vi "SDT_GenerateMeasureInfoBlockDecayCurves.vi"(4 "EndTimeArray":dbl[](array[numeric]), 8 "ActiveModule":string[](array[string]), 9 "DecayMatrix":u32[][](array[numeric]), 10 "Module Type":T12 items=["SPC-600"=600, "SPC-630"=630, "SPC-700"=700, "SPC-730"=730, "SPC-130"=130, "SPC-830"=830, "SPC-140"=140, "SPC-930"=930, "DPC-230"=230, "SPC-150"=150, "SPC-150 N"=151, "SPC-150 NX"=152, "SPC-130 EM"=131, "SPC-130 EMN"=132, "SPC-130IN"=135, "SPC-130INX"=136, "SPC-130INXX"=137, "SPC-160"=160, "SPC-160 X"=161, "SPC-160 PCIE"=162, "SPC-180 N"=180, "SPC-180 NX"=181, "SPC-180 NXX"=182, "SPC-180 N-USB"=185, "SPC-180 NX-USB"=186, "SPC-180 NXX-USB"=187, "SPC-QC-104"=104, "SPC-QC-004"=4, "SPC-QC-106"=106, "DPC-330"=330, "PMS-800"=800, "SPC-590"=590, "Simulation"=-1], 11 "SPCdata":T11[](array[typedef])) -> (2 "MeasureInfoStrings":string[](array[string]), 3 "MeasureInfos":T1[](array[typedef]) {"MeasStopInfo"."flags" format="x%x"})   [LabVIEW 2017]
doc: "This VI is a SubVI to SDT_WriteFile.vi. It populates the arrays of MeasureInfos cluster and generates strings ready to be written to file. \nFor a description of the *.sdt file format see: SPC_data_file_structure.h\n\ninfo@becker-hickl.com"
uses:
  SPC_Wrappers/SPC_Controls/ModuleType.ctl
  SPC_Wrappers/SPC_Controls/SPCdata.ctl
  SPC_Wrappers/SPC_Controls/MeasureInfo.ctl
  SPC_Wrappers/SPC_Controls/MeasureInfo_PartB.ctl
  SPC_Wrappers/SPC_Controls/MeasStopInfo.ctl
  SPC_Wrappers/SPC_Controls/MeasFCSInfo.ctl
  SPC_Wrappers/SPC_Controls/MeasureInfo_PartE.ctl
  SPC_Wrappers/SPC_Controls/MeasHISTInfo.ctl
  SPC_Wrappers/SPC_Controls/HISTInfoExt.ctl
  SPC_Wrappers/SPC_Controls/MeasureInfo_PartI.ctl
  SPC_Wrappers/SPC_Controls/MeasureInfo_PartK.ctl
  SPC_Wrappers/SPC_Controls/MeasureInfo_PartM.ctl
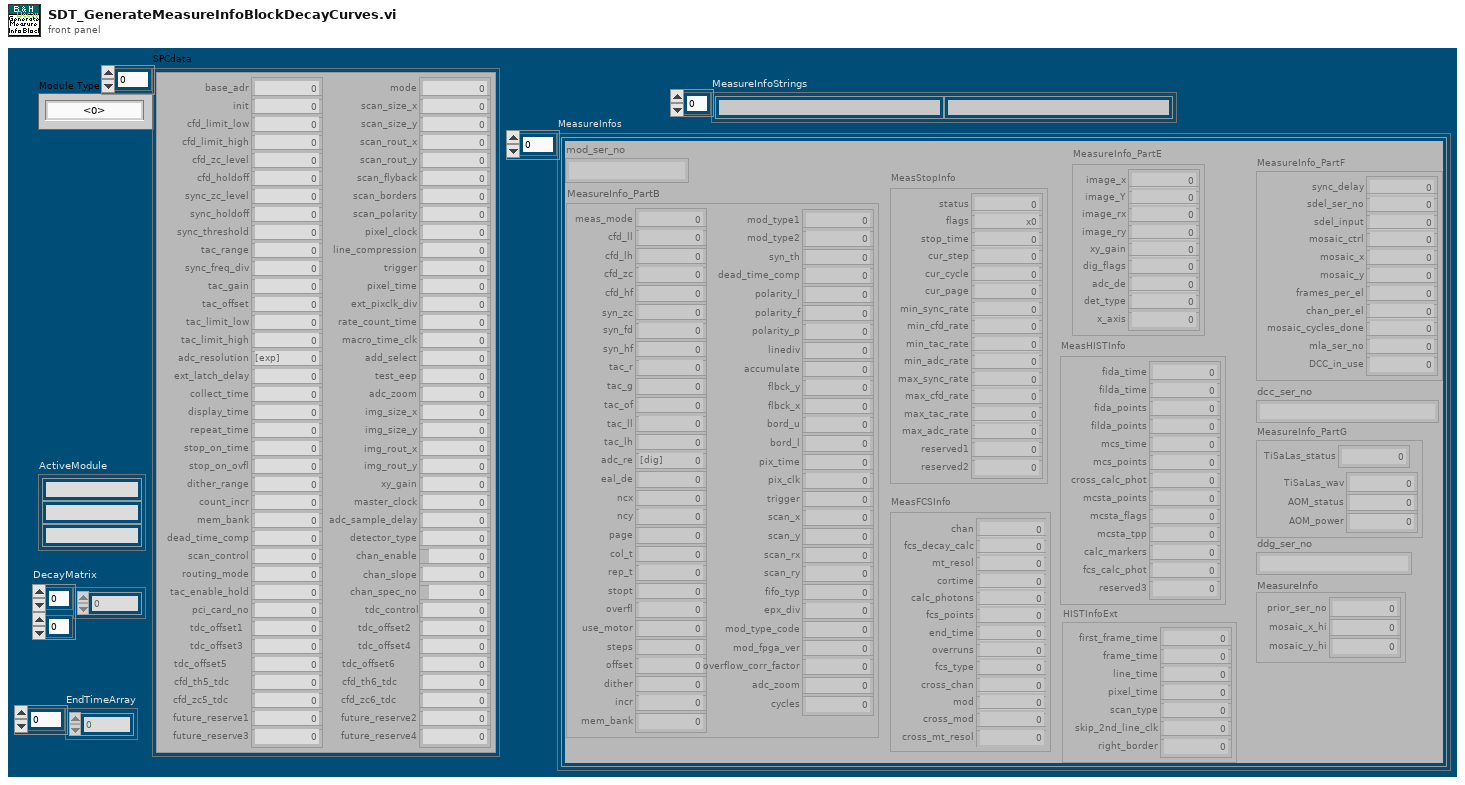
[diagram p1: front panel]
types:
  T1 = typedef "MeasureInfo.ctl" = cluster{"mod_ser_no":string, "MeasureInfo_PartB":T2, "MeasStopInfo":T3, "MeasFCSInfo":T4, "MeasureInfo_PartE":T5, "MeasHISTInfo":T6, "HISTInfoExt":T7, "MeasureInfo_PartF":T8, "dcc_ser_no":string, "MeasureInfo_PartG":T9, "ddg_ser_no":string, "MeasureInfo":T10}
  T2 = typedef "MeasureInfo_PartB.ctl" = cluster{"meas_mode":i16, "cfd_ll":sgl, "cfd_lh":sgl, "cfd_zc":sgl, "cfd_hf":sgl, "syn_zc":sgl, "syn_fd":i16, "syn_hf":sgl, "tac_r":sgl, "tac_g":i16, "tac_of":sgl, "tac_ll":sgl, "tac_lh":sgl, "adc_re":i16, "eal_de":i16, "ncx":i16, "ncy":i16, "page":u16, "col_t":sgl, "rep_t":sgl, "stopt":i16, "overfl":i8, "use_motor":i16, "steps":u16, "offset":sgl, "dither":i16, "incr":i16, "mem_bank":i16, "mod_type1":u64, "mod_type2":u64, "syn_th":sgl, "dead_time_comp":i16, "polarity_l":i16, "polarity_f":i16, "polarity_p":i16, "linediv":i16, "accumulate":i16, "flbck_y":i32, "flbck_x":i32, "bord_u":i32, "bord_l":i32, "pix_time":sgl, "pix_clk":i16, "trigger":i16, "scan_x":i32, "scan_y":i32, "scan_rx":i32, "scan_ry":i32, "fifo_typ":i16, "epx_div":i32, "mod_type_code":u16, "mod_fpga_ver":u16, "overflow_corr_factor":sgl, "adc_zoom":i32, "cycles":i32}
  T3 = typedef "MeasStopInfo.ctl" = cluster{"status":u16, "flags":u16, "stop_time":sgl, "cur_step":i32, "cur_cycle":i32, "cur_page":i32, "min_sync_rate":sgl, "min_cfd_rate":sgl, "min_tac_rate":sgl, "min_adc_rate":sgl, "max_sync_rate":sgl, "max_cfd_rate":sgl, "max_tac_rate":sgl, "max_adc_rate":sgl, "reserved1":i32, "reserved2":sgl}
  T4 = typedef "MeasFCSInfo.ctl" = cluster{"chan":u16, "fcs_decay_calc":u16, "mt_resol":u32, "cortime":sgl, "calc_photons":u32, "fcs_points":i32, "end_time":sgl, "overruns":u16, "fcs_type":u16, "cross_chan":u16, "mod":u16, "cross_mod":u16, "cross_mt_resol":u32}
  T5 = typedef "MeasureInfo_PartE.ctl" = cluster{"image_x":i32, "image_Y":i32, "image_rx":i32, "image_ry":i32, "xy_gain":i16, "dig_flags":i16, "adc_de":i16, "det_type":i16, "x_axis":i16}
  T6 = typedef "MeasHISTInfo.ctl" = cluster{"fida_time":sgl, "filda_time":sgl, "fida_points":i32, "filda_points":i32, "mcs_time":sgl, "mcs_points":i32, "cross_calc_phot":u32, "mcsta_points":u16, "mcsta_flags":u16, "mcsta_tpp":u32, "calc_markers":u32, "fcs_calc_phot":u32, "reserved3":u32}
  T7 = typedef "HISTInfoExt.ctl" = cluster{"first_frame_time":sgl, "frame_time":sgl, "line_time":sgl, "pixel_time":sgl, "scan_type":i16, "skip_2nd_line_clk":i16, "right_border":u32}
  T8 = typedef "MeasureInfo_PartI.ctl" = cluster{"sync_delay":sgl, "sdel_ser_no":u16, "sdel_input":i8, "mosaic_ctrl":i8, "mosaic_x":u8, "mosaic_y":u8, "frames_per_el":i16, "chan_per_el":i16, "mosaic_cycles_done":i32, "mla_ser_no":u16, "DCC_in_use":u8}
  T9 = typedef "MeasureInfo_PartK.ctl" = cluster{"TiSaLas_status":u16, "TiSaLas_wav":u16, "AOM_status":u8, "AOM_power":u8}
  T10 = typedef "MeasureInfo_PartM.ctl" = cluster{"prior_ser_no":i32, "mosaic_x_hi":u8, "mosaic_y_hi":u8}
  T11 = typedef "SPCdata.ctl" = cluster{"base_adr":u16, "init":i16, "cfd_limit_low":sgl, "cfd_limit_high":sgl, "cfd_zc_level":sgl, "cfd_holdoff":sgl, "sync_zc_level":sgl, "sync_holdoff":sgl, "sync_threshold":sgl, "tac_range":sgl, "sync_freq_div":i16, "tac_gain":i16, "tac_offset":sgl, "tac_limit_low":sgl, "tac_limit_high":sgl, "adc_resolution":i16, "ext_latch_delay":i16, "collect_time":sgl, "display_time":sgl, "repeat_time":sgl, "stop_on_time":i16, "stop_on_ovfl":i16, "dither_range":i16, "count_incr":i16, "mem_bank":i16, "dead_time_comp":i16, "scan_control":u16, "routing_mode":u16, "tac_enable_hold":sgl, "pci_card_no":i16, "mode":u16, "scan_size_x":u32, "scan_size_y":u32, "scan_rout_x":u32, "scan_rout_y":u32, "scan_flyback":u32, "scan_borders":u32, "scan_polarity":u16, "pixel_clock":u16, "line_compression":u16, "trigger":u16, "pixel_time":sgl, "ext_pixclk_div":u32, "rate_count_time":sgl, "macro_time_clk":i16, "add_select":i16, "test_eep":i16, "adc_zoom":i16, "img_size_x":u32, "img_size_y":u32, "img_rout_x":u32, "img_rout_y":u32, "xy_gain":i16, "master_clock":i16, "adc_sample_delay":i16, "detector_type":i16, "chan_enable":u32, "chan_slope":u32, "chan_spec_no":u32, "tdc_control":u32, "tdc_offset1":sgl, "tdc_offset2":sgl, "tdc_offset3":sgl, "tdc_offset4":sgl, "tdc_offset5":sgl, "tdc_offset6":sgl, "cfd_th5_tdc":sgl, "cfd_th6_tdc":sgl, "cfd_zc5_tdc":sgl, "cfd_zc6_tdc":sgl, "future_reserve1":u64, "future_reserve2":u64, "future_reserve3":u64, "future_reserve4":u64}
  T12 = typedef "ModuleType.ctl" = i16
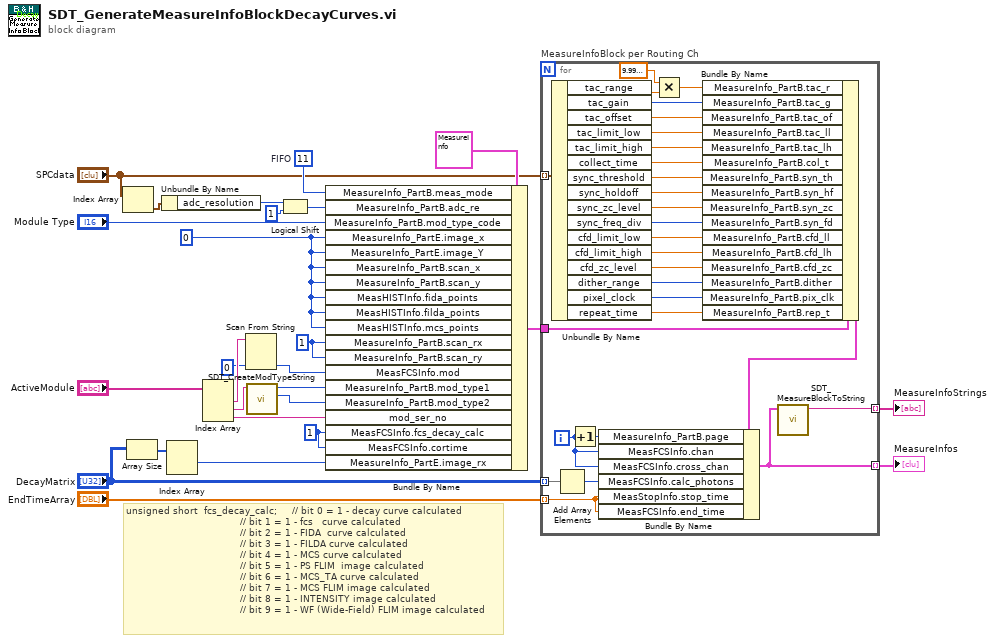
[diagram p0: block diagram]
diagram:
  w8 = i16 11  # FIFO
  w6 = u16 1 ("MeasFCSInfo.fcs_decay_calc")
  w11 = 0 ("ImageSize")
  w21 = 1 ("MeasureInfo_PartB.scan_rx")
  # "unsigned short  fcs_decay_calc;     // bit 0 = 1 - decay curve calculated\n                                      // bit 1 = 1 - fcs   curve calculated\n                                      // bit 2 = 1 - FIDA  curve calculated\n                                      // bit 3 = 1 - FILDA curve calculated\n                                      // bit 4 = 1 - MCS curve calculated\n                                      // bit 5 = 1 - PS FLIM  image calculated\n                                      // bit 6 = 1 - MCS_TA curve calculated\n                                      // bit 7 = 1 - MCS FLIM image calculated\n                                      // bit 8 = 1 - INTENSITY image calculated\n                                      // bit 9 = 1 - WF (Wide-Field) FLIM image calculated"
  n1 = Index Array(array="SPCdata") -> (element=w4:T11)  [unwired: 1 in]
  n2 = Array Size(array="DecayMatrix") -> (size(s)=w17:i32[])
  n3 = Unbundle By Name(w4) -> ("adc_resolution"=w2:i16)
  n4 = Index Array(array=w17) -> (element #1=w16:i32)  [unwired: 2 in, 1 out]
  n5 = Index Array(array="ActiveModule") -> (element #1=w20:string, element #2=w26:string, element #3=w24:string)  [unwired: 3 in]
  n6 = Scan From String(input string=w20, default 1=u16 0 ("meas_desc_block_no")) -> (output 1=w18:u16)  [unwired: 3 in, 3 out]
  n7 = call "SDT_CreateModTypeString.vi"("mod_type-String"=w26) -> ("mod_type2"=w23:u64, "mod_type1"=w22:u64)  [unwired: 9 in]
  n8 = Logical Shift(y=w2, x=u32 1) -> (x << y=w1:u32)
  n9 = Bundle By Name(cluster=T1 {"mod_ser_no"="3F0024\u0000\u0000\u0000\u0000\u0000\u0000\u0000\u0000\u0000\u0000", "MeasureInfo_PartB"={"meas_mode"=13, "cfd_ll"=-29.411764, "cfd_lh"=5.019608, "cfd_zc"=12.850393, "cfd_hf"=5.0, "syn_zc"=-5.2913384, "syn_fd"=1, "syn_hf"=4.0, "tac_r"=5.0033574e-08, "tac_g"=3, "tac_of"=7.45098, "tac_ll"=5.098039, "tac_lh"=95.29412, "adc_re"=4096, "eal_de"=0, "ncx"=1, "ncy"=1, "page"=1, "col_t"=20.0, "rep_t"=20.0, "stopt"=0, "overfl"=78, "use_motor"=0, "steps"=1, "offset"=0.0, "dither"=128, "incr"=1, "mem_bank"=0, "mod_type1"=13570383722795091, "mod_type2"=0, "syn_th"=-50.980392, "dead_time_comp"=0, "polarity_l"=1, "polarity_f"=1, "polarity_p"=1, "linediv"=0, "accumulate"=0, "flbck_y"=1, "flbck_x"=1, "bord_u"=0, "bord_l"=0, "pix_time"=2e-07, "pix_clk"=1, "trigger"=16, "scan_x"=256, "scan_y"=256, "scan_rx"=1, "scan_ry"=1, "fifo_typ"=0, "epx_div"=1, "mod_type_code"=160, "mod_fpga_ver"=514, "overflow_corr_factor"=0.0, "adc_zoom"=0, "cycles"=1}, "MeasStopInfo"={"status"=824, "flags"=33199, "stop_time"=377.24805, "cur_step"=1, "cur_cycle"=1, "cur_page"=1, "min_sync_rate"=12634368.0, "min_cfd_rate"=1056.0, "min_tac_rate"=1056.0, "min_adc_rate"=70432.0, "max_sync_rate"=40678656.0, "max_cfd_rate"=769936.0, "max_tac_rate"=581984.0, "max_adc_rate"=565856.0, "reserved1"=0, "reserved2"=0.0}, "MeasFCSInfo"={"chan"=1, "fcs_decay_calc"=32, "mt_resol"=250, "cortime"=1.0, "calc_photons"=164220395, "fcs_points"=0, "end_time"=377.2369, "overruns"=0, "fcs_type"=32801, "cross_chan"=8, "mod"=0, "cross_mod"=0, "cross_mt_resol"=250}, "MeasureInfo_PartE"={"image_x"=256, "image_Y"=256, "image_rx"=1, "image_ry"=1, "xy_gain"=0, "dig_flags"=0, "adc_de"=0, "det_type"=0, "x_axis"=0}, "MeasHISTInfo"={"fida_time"=0.0, "filda_time"=0.0, "fida_points"=258, "filda_points"=512, "mcs_time"=0.0, "mcs_points"=512, "cross_calc_phot"=0, "mcsta_points"=0, "mcsta_flags"=0, "mcsta_tpp"=0, "calc_markers"=0, "fcs_calc_phot"=0, "reserved3"=0}, "HISTInfoExt"={"first_frame_time"=0.10108537, "frame_time"=1.4619007, "line_time"=0.002849475, "pixel_time"=4.4e-06, "scan_type"=0, "skip_2nd_line_clk"=0, "right_border"=0}, "MeasureInfo_PartF"={"sync_delay"=0.0, "sdel_ser_no"=0, "sdel_input"=0, "mosaic_ctrl"=0, "mosaic_x"=4, "mosaic_y"=4, "frames_per_el"=2, "chan_per_el"=1, "mosaic_cycles_done"=0, "mla_ser_no"=0, "DCC_in_use"=17}, "dcc_ser_no"="8A0043\u0000\u0000\u0000\u0000\u0000\u0000", "MeasureInfo_PartG"={"TiSaLas_status"=0, "TiSaLas_wav"=0, "AOM_status"=0, "AOM_power"=0}, "ddg_ser_no"="\u0000\u0000\u0000\u0000\u0000\u0000\u0000\u0000", "MeasureInfo"={"prior_ser_no"=0, "mosaic_x_hi"=0, "mosaic_y_hi"=0}} ("MeasureInfo"), "MeasureInfo_PartB.meas_mode"=w8, "MeasureInfo_PartB.adc_re"=w1, "MeasureInfo_PartB.mod_type_code"="Module Type", "MeasureInfo_PartE.image_x"=w11, "MeasureInfo_PartE.image_Y"=w11, "MeasureInfo_PartB.scan_x"=w11, "MeasureInfo_PartB.scan_y"=w11, "MeasHISTInfo.fida_points"=w11, "MeasHISTInfo.filda_points"=w11, "MeasHISTInfo.mcs_points"=w11, "MeasureInfo_PartB.scan_rx"=w21, "MeasureInfo_PartB.scan_ry"=w21, "MeasFCSInfo.mod"=w18, "MeasureInfo_PartB.mod_type1"=w22, "MeasureInfo_PartB.mod_type2"=w23, "mod_ser_no"=w24, "MeasFCSInfo.fcs_decay_calc"=w6, "MeasFCSInfo.cortime"=w6, "MeasureInfo_PartE.image_rx"=w16) -> (w9:T1)
  n10 = for "MeasureInfoBlock per Routing Ch" {
    tunnel: "DecayMatrix" -> [w54] mode=indexing
    tunnel: [w52] -> w15 mode=indexing
    tunnel: [w51] -> w14 mode=indexing
    tunnel: w9 -> [w33]
    tunnel: "SPCdata" -> [w32] mode=indexing
    tunnel: "EndTimeArray" -> [w30] mode=indexing
    i -> [w29]
    n11 = Unbundle By Name(w32) -> ("tac_range"=w50:sgl, "tac_gain"=w47:i16, "tac_offset"=w46:sgl, "tac_limit_low"=w45:sgl, "tac_limit_high"=w44:sgl, "collect_time"=w43:sgl, "sync_threshold"=w42:sgl, "sync_holdoff"=w41:sgl, "sync_zc_level"=w40:sgl, "sync_freq_div"=w39:i16, "cfd_limit_low"=w38:sgl, "cfd_limit_high"=w37:sgl, "cfd_zc_level"=w36:sgl, "dither_range"=w35:i16, "pixel_clock"=w34:u16, "repeat_time"=w27:sgl)
    n12 = Add Array Elements(numeric array=w54) -> (sum=w53:u32)
    n13 = Increment(x=w29) -> (x+1=w28:i32)
    n14 = Multiply(x=sgl 1e-09 ("y"), y=w50) -> (x*y=w48:sgl)
    n15 = Bundle By Name(cluster=w33, "MeasureInfo_PartB.tac_r"=w48, "MeasureInfo_PartB.tac_g"=w47, "MeasureInfo_PartB.tac_of"=w46, "MeasureInfo_PartB.tac_ll"=w45, "MeasureInfo_PartB.tac_lh"=w44, "MeasureInfo_PartB.col_t"=w43, "MeasureInfo_PartB.syn_th"=w42, "MeasureInfo_PartB.syn_hf"=w41, "MeasureInfo_PartB.syn_zc"=w40, "MeasureInfo_PartB.syn_fd"=w39, "MeasureInfo_PartB.cfd_ll"=w38, "MeasureInfo_PartB.cfd_lh"=w37, "MeasureInfo_PartB.cfd_zc"=w36, "MeasureInfo_PartB.dither"=w35, "MeasureInfo_PartB.pix_clk"=w34, "MeasureInfo_PartB.rep_t"=w27) -> (w31:T1)
    n16 = Bundle By Name(cluster=w31, "MeasureInfo_PartB.page"=w28, "MeasFCSInfo.chan"=w29, "MeasFCSInfo.cross_chan"=w29, "MeasFCSInfo.calc_photons"=w53, "MeasStopInfo.stop_time"=w30, "MeasFCSInfo.end_time"=w30) -> (w52:T1)
    n17 = call "SDT_MeasureBlockToString.vi"("MeasureInfo"=w52) -> ("MeasureBlockString"=w51:string)  [unwired: 9 in, 1 out]
  }
  "MeasureInfos" <- w15
  "MeasureInfoStrings" <- w14
